vi "Main.vi"(11 "Module Admin":refnum<class "Delacor_lib_QMH_Module Admin.lvclass">) -> ()   [LabVIEW 2019, in "ContextHelp.lvlib"]
doc: "This template is based off of the Queued Message Handler design pattern and the Queued Message Handler project template that ships with LabVIEW.\n\nThe main difference is that the queue is private to this module and communication between modules is performed via Broadcast and Request events.\n\nRequest events are wrapped in public API methods and are handled in the Event Handling Loop (EHL) of this VI. Any module can register for Broadcast events sent by this module. The EHL generates messages based on user interface actions.\n\nThe Message Handling Loop (MHL) processes messages generated by the EHL, or by other messages. The messages are string values, so new messages can be added easily to the Message Cases case structure in the MHL. Each message cluster can also provide an optional value for Message Data, which is a variant that can be converted to whatever message-specific data is required.\n_____\nBased on DQMH Project Template 6.1.0.94.\n____\nPantherLAB Templates 1.0.0.5\nCopyright (c) 2022, PantherLAB"
uses:
  ContextHelp.lvlib
  <vilib>/Delacor/Delacor QMH/Libraries/Module Admin_class/Delacor_lib_QMH_Module Admin.lvclass
  Module Data--cluster.ctl
  <vilib>/Delacor/Delacor QMH/Libraries/Message Queue_class/Delacor_lib_QMH_Message Queue.lvclass/Delacor_lib_QMH_Message Queue.ctl
  Stop Argument--cluster.ctl
  <vilib>/Delacor/Delacor QMH/Libraries/Module Admin_class/Delacor_lib_QMH_Module Admin.lvclass/Delacor_lib_QMH_Module Admin.ctl
  Draw Panel Into Subpanel Argument--cluster.ctl
  Remove Panel from Subpanel Argument--cluster.ctl
  <vilib>/Delacor/Delacor QMH/Libraries/Message Queue_class/Delacor_lib_QMH_Enqueue Message (Single).vi
  <vilib>/Delacor/Delacor QMH/Libraries/Module Admin_class/Delacor_lib_QMH_Get External Launch.vi
  <vilib>/Utility/error.llb/Error Cluster From Error Code.vi
  <vilib>/ErrorRing/Error Ring.xnode
  <vilib>/Delacor/Delacor QMH/Libraries/Message Queue_class/Delacor_lib_QMH_Message Queue.lvclass
  Panther Dashboard/Panther Dashboard.lvlib
  Shared/Shared.lvlib
panel:
  out "Status":string
  out "error out":errorcluster
  in  "Edit Project Description":bool caption="Project Documentation"
  in  "Project Description":string
  in  "Edit Module Description":bool caption="Module Description"
  in  "Module Description":string
  in  "Edit VI":bool caption="Event Description"
  out "Event Connector Pane":picture
  in  "Event Description":string
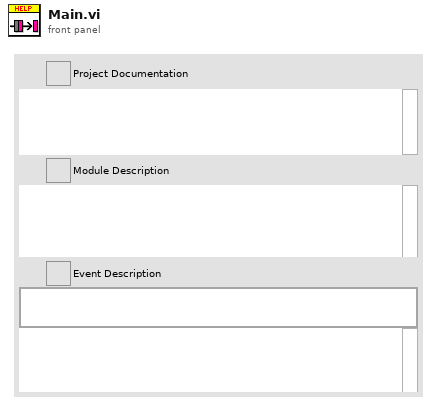
[diagram p1: front panel]
types:
  T1 = typedef "Panther Dashboard.lvlib/Broadcast Events--cluster.ctl" = cluster{"Module Did Init":refnum<user-event>, "Status Updated":refnum<user-event>, "Error Reported":refnum<user-event>, "Module Did Stop":refnum<user-event>, "Update Module Execution Status":refnum<user-event>, "References Updated":refnum<user-event>, "Projects Updated":refnum<user-event>, "Targets Updated":refnum<user-event>, "Progress updated":refnum<user-event>, "Scale Updated":refnum<user-event>, "Connector Pane Updated":refnum<user-event>, "Documentation Updated":refnum<user-event>, "Module Type Updated":refnum<user-event>, "Theme Updated":refnum<user-event>, "Project Description Updated":refnum<user-event>}
  T2 = typedef "ContextHelp.lvlib/Request Events--cluster.ctl" = cluster{"Stop Module":refnum<user-event>, "Show Panel":refnum<user-event>, "Hide Panel":refnum<user-event>, "Get Module Execution Status":refnum<user-event>, "Show Diagram":refnum<user-event>, "Wake up Helper Loop":refnum<user-event>, "Put Helper Loop to Sleep":refnum<user-event>, "Draw Panel Into Subpanel":refnum<user-event>, "Remove Panel from Subpanel":refnum<user-event>, "Refresh Panther Dashboard Broadcasts":refnum<user-event>}
  T3 = typedef "ContextHelp.lvlib/Module Data--cluster.ctl" = cluster{"Status":string, "SubPanel":refnum<vi>, "Panel Status":bool}
  T4 = enum8{"Enabled", "Disabled", "Disabled and Grayed Out"}
  T5 = enum32{"invalid lock state", "Not Locked", "Locked (No Password)", "Password-protected"}
  T6 = typedef "ContextHelp.lvlib/Stop Argument--cluster.ctl" = cluster{"Origin":string, "Exit via Stop Module Req?":bool, "Wait for Module to stop?":bool}
  T7 = typedef "ContextHelp.lvlib/Draw Panel Into Subpanel Argument--cluster.ctl" = cluster{"Sub Panel":refnum<vi>}
  T8 = typedef "ContextHelp.lvlib/Remove Panel from Subpanel Argument--cluster.ctl" = cluster{"Boolean":bool}
  T9 = enum32{"Invalid", "Standard", "Closed", "Hidden", "Minimized", "Maximized"}
  T10 = typedef "LVRectTypeDef.ctl" = cluster{"Left":i16, "Top":i16, "Right":i16, "Bottom":i16}
  T11 = typedef "Panther Dashboard.lvlib/Documentation--cluster.ctl" = cluster{"Module Description":string, "Event Description":string}
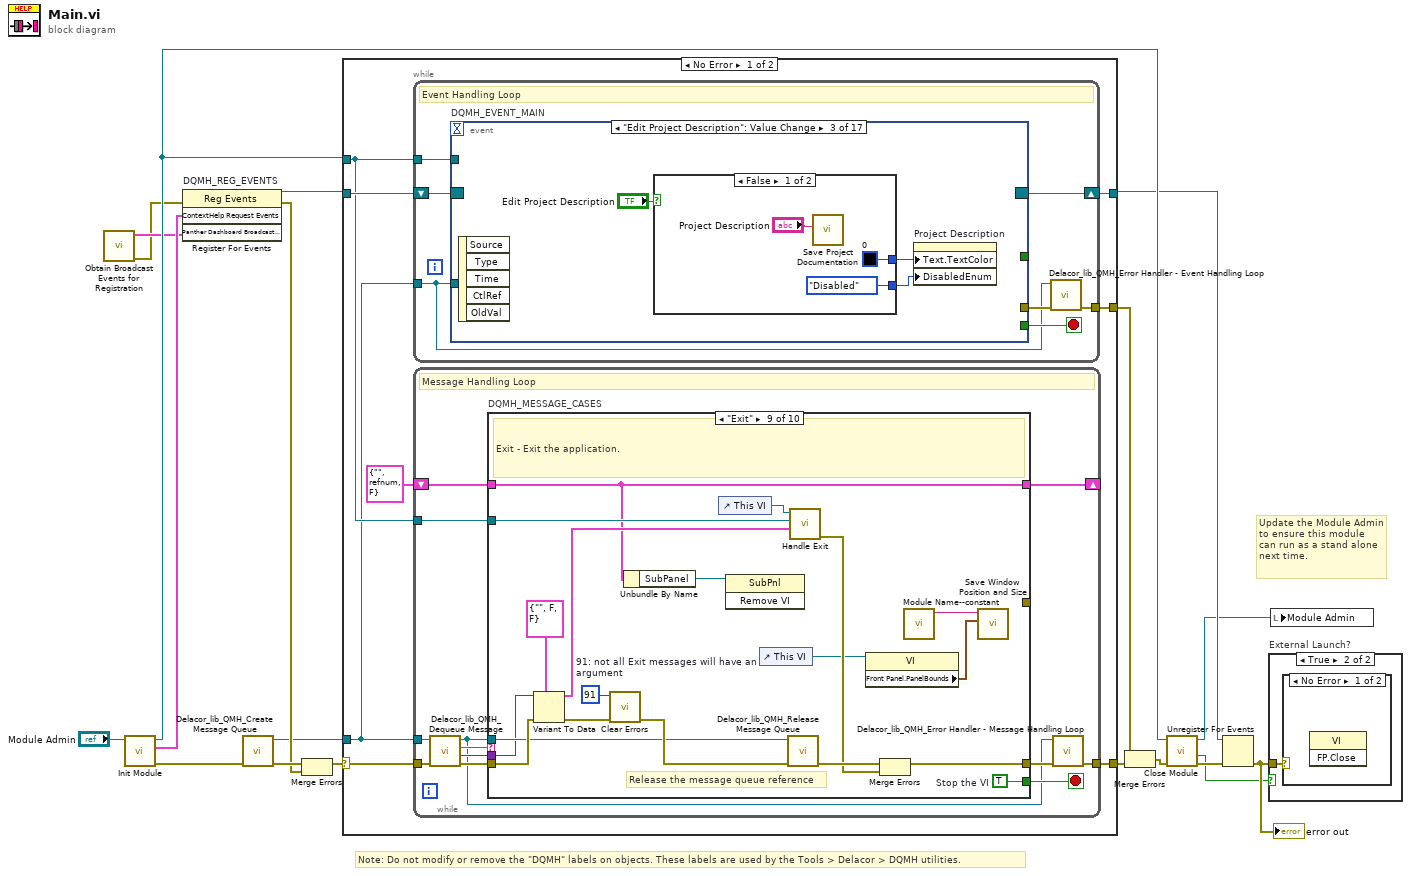
[diagram p0: block diagram]
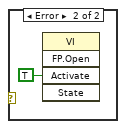
[diagram p3: hidden frame]
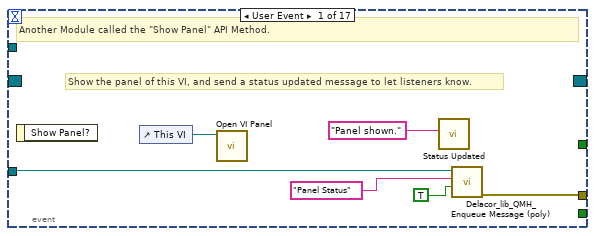
[diagram p4: hidden frame]
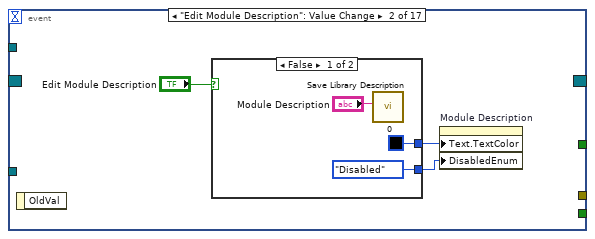
[diagram p5: hidden frame]
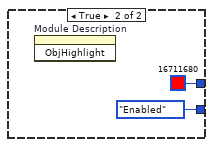
[diagram p6: hidden frame]
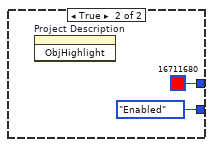
[diagram p7: hidden frame]
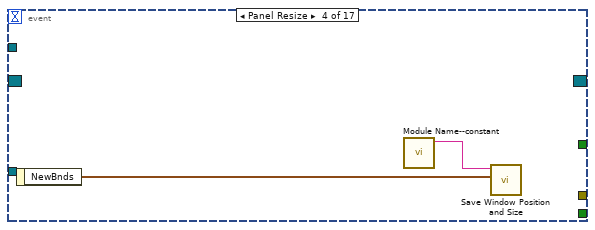
[diagram p8: hidden frame]
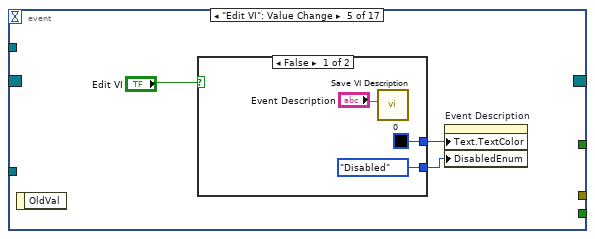
[diagram p9: hidden frame]
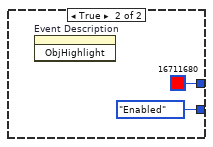
[diagram p10: hidden frame]
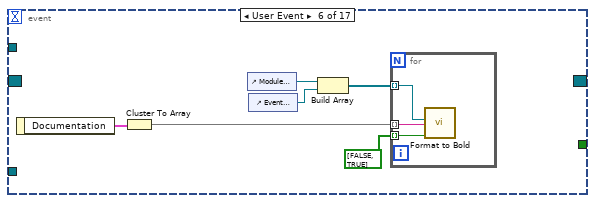
[diagram p11: hidden frame]
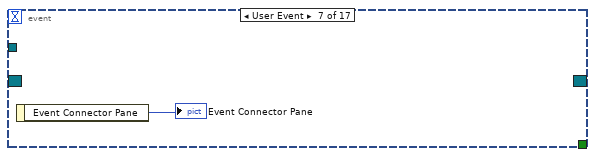
[diagram p12: hidden frame]
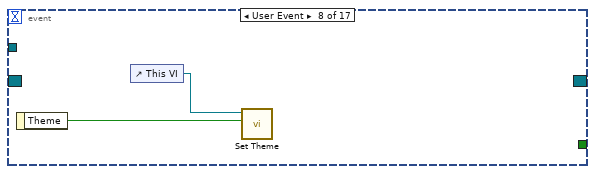
[diagram p13: hidden frame]
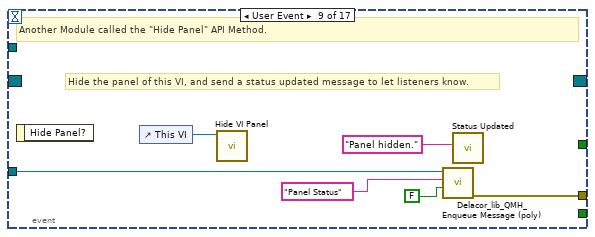
[diagram p14: hidden frame]
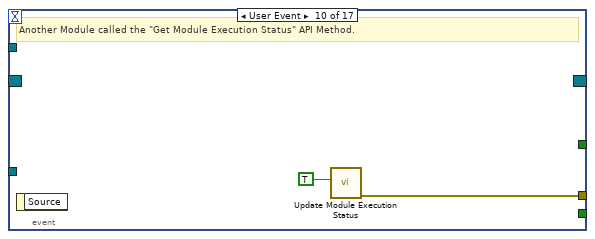
[diagram p15: hidden frame]
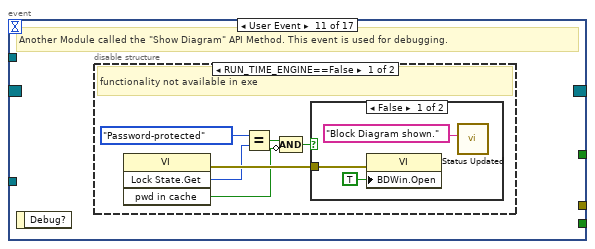
[diagram p16: hidden frame]
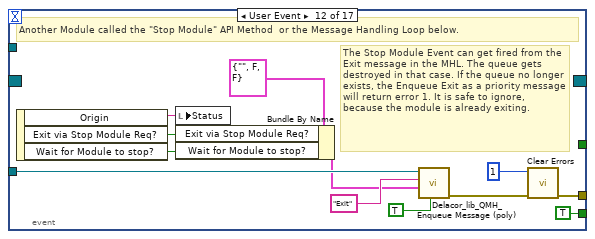
[diagram p19: hidden frame]
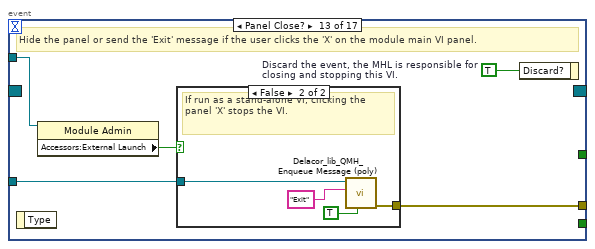
[diagram p20: hidden frame]
diagram:
  # "Note: Do not modify or remove the \"DQMH\" labels on objects. These labels are used by the Tools > Delacor > DQMH utilities."
  # "Update the Module Admin to ensure this module can run as a stand alone next time."
  n1 = call "Obtain Broadcast Events for Registration.vi"() -> ("error out"=w1:errorcluster, "Panther Dashboard Broadcast Events"=w2:T1)  [unwired: 9 in, 1 out]
  n2 = call "Init Module.vi"("Singleton Module Admin in"="Module Admin") -> ("error out"=w18:errorcluster, "ContextHelp Request Events"=w3:T2, "Singleton Module Admin out"=w10:refnum<class "Delacor_lib_QMH_Module Admin.lvclass">)  [unwired: 8 in]
  n3 = register-events "DQMH_REG_EVENTS"(error in=w1, w3, w2) -> (reference out=w8:refnum<event-registration>, error out=w11:errorcluster)  [unwired: 1 in]
  n4 = call <vilib>:"Delacor_lib_QMH_Create Message Queue.vi"("error in"=w18) -> ("error out"=w13:errorcluster, "Message Queue"=w7:refnum<class "Delacor_lib_QMH_Message Queue.lvclass">)  [unwired: 9 in]
  n5 = Merge Errors(w13, w11) -> (w12:errorcluster)
  n6 = case shown="No Error" w12 {
    selector: w12 -> [w25 w261]
    tunnel: [w27 w260] -> w19
    tunnel: [w24 w259] -> w9
    tunnel: w8 -> [w22 w259]
    tunnel: w7 -> [w20 w254]
    tunnel: [w26 _] -> w16
    tunnel: w10 -> [w21 w255]
    frame No Error {
      n7 = while {
        tunnel: w20 -> [w28]
        shift-right: [w31] -> w24
        shift-left: w22 -> [w32]
        tunnel: [w33] -> w26
        tunnel: w21 -> [w29]
        stop <- w30 stop-if-true
        # "Event Handling Loop"
        n8 = event "DQMH_EVENT_MAIN" shown="[2] \"Edit Project Description\": Value Change" {
          selector: w32 -> [_ _ _ _ _ _ _ _ _ _ _ _ _ _ _ w133 _]
          dyn-events: [_ _ _ _ _ _ _ _ _ _ _ _ _ _ _ w132 _] -> w31
          timeout: _ -> [_ _ _ _ _ _ _ _ _ _ _ _ _ _ _ _ _]
          tunnel: [_ _ _ _ _ _ _ _ _ _ _ TRUE ("Discard?") _ _ _ _ _] -> w30
          tunnel: w28 -> [w37 _ _ _ _ _ _ _ w79 _ _ w103 w110 w122 w128 _ _]
          tunnel: [w40 _ _ _ _ _ _ _ w84 w86 _ w106 w112 w123 w129 _ _] -> w34
          tunnel: w29 -> [_ _ _ _ _ _ _ _ _ _ _ _ w109 _ _ _ _]
          tunnel: [_ _ _ _ _ _ _ _ _ _ _ _ _ _ _ w130 _] -> _
          event User Event {
            # "Show the panel of this VI, and send a status updated message to let listeners know."
            # "Another Module called the \"Show Panel\" API Method."
            n9 = event-data() -> ()  [unwired: 1 in, 1 out]
            n10 = control-ref of="This VI"() -> (w39:refnum<vi>)
            n11 = call "Open VI Panel.vi"("VI"=w39) -> ()  [unwired: 10 in, 1 out]
            n12 = call "Status Updated.vi"("Status"="Panel shown." ("format string")) -> ()  [unwired: 10 in, 1 out]
            n13 = call-poly <vilib>:"Delacor_lib_QMH_Enqueue Message (poly).vi"("Message Data"=TRUE, "Message"="Panel Status" ("format string"), "Message Queue in"=w37) -> ("error out"=w40:errorcluster)  [unwired: 7 in, 1 out]
          }
          event "Edit Module Description": Value Change {
            n14 = event-data() -> ()  [unwired: 1 in, 1 out]
            n15 = case shown="False" "Edit Module Description" {
              tunnel: [u32 0 u32 16711680] -> w42
              tunnel: [T4."Disabled" ("Disabled") T4."Enabled" ("Disabled")] -> w43
              frame False {
                n16 = call "Save Library Description.vi"("Library Description"="Module Description") -> ()  [unwired: 10 in, 1 out]
              }
              frame True {
                n17 = invoke on="Module Description" class="Str" method="ObjHighlight"() -> ()  [unwired: 3 in, 3 out]
              }
            }
            n18 = property on="Module Description" class="Str"("Text.TextColor"=w42, "DisabledEnum"=w43) -> ()  [unwired: 2 in, 2 out]
          }
          event "Edit Project Description": Value Change {
            n19 = event-data() -> ()  [unwired: 1 in, 5 out]
            n20 = case shown="False" "Edit Project Description" {
              tunnel: [u32 0 u32 16711680] -> w50
              tunnel: [T4."Disabled" ("Disabled") T4."Enabled" ("Disabled")] -> w51
              frame False {
                n21 = call "Save Project Documentation.vi"("Project Description"="Project Description") -> ()  [unwired: 10 in, 1 out]
              }
              frame True {
                n22 = invoke on="Project Description" class="Str" method="ObjHighlight"() -> ()  [unwired: 3 in, 3 out]
              }
            }
            n23 = property on="Project Description" class="Str"("Text.TextColor"=w50, "DisabledEnum"=w51) -> ()  [unwired: 2 in, 2 out]
          }
          event Panel Resize {
            n24 = event-data() -> ("NewBnds"=w58:T10)  [unwired: 1 in]
            n25 = call "Module Name--constant.vi"() -> ("Module Name"=w57:string)  [unwired: 11 in]
            n26 = call "Save Window Position and Size.vi"("NewBnds"=w58, "Position Key"=w57) -> ()  [unwired: 9 in, 1 out]
          }
          event "Edit VI": Value Change {
            n27 = event-data() -> ()  [unwired: 1 in, 1 out]
            n28 = case shown="False" "Edit VI" {
              tunnel: [u32 0 u32 16711680] -> w60
              tunnel: [T4."Disabled" ("Disabled") T4."Enabled" ("Disabled")] -> w61
              frame False {
                n29 = call "Save VI Description.vi"("VI Description"="Event Description") -> ()  [unwired: 10 in, 1 out]
              }
              frame True {
                n30 = invoke on="Event Description" class="Str" method="ObjHighlight"() -> ()  [unwired: 3 in, 3 out]
              }
            }
            n31 = property on="Event Description" class="Str"("Text.TextColor"=w60, "DisabledEnum"=w61) -> ()  [unwired: 2 in, 2 out]
          }
          event User Event {
            n32 = event-data() -> ("Documentation"=w72:T11)  [unwired: 1 in]
            n33 = Cluster To Array(cluster=w72) -> (array=w70:string[])
            n34 = control-ref of="Module Description"() -> (w68:refnum<vi>)
            n35 = control-ref of="Event Description"() -> (w67:refnum<vi>)
            n36 = Build Array(w68, w67) -> (w69:refnum<vi>[])
            n37 = for {
              tunnel: bool[] [FALSE, TRUE] ("Adjust Height?") -> [w75] mode=indexing
              tunnel: w70 -> [w74] mode=indexing
              tunnel: w69 -> [w73] mode=indexing
              n38 = call "Format to Bold.vi"("Adjust Height?"=w75, "String Value"=w74, "String Ref"=w73) -> ()  [unwired: 9 in]
            }
          }
          event User Event {
            n39 = event-data() -> ("Event Connector Pane"=→"Event Connector Pane":picture)  [unwired: 1 in]
          }
          event User Event {
            n40 = event-data() -> ("Theme"=w77:bool)  [unwired: 1 in]
            n41 = control-ref of="This VI"() -> (w78:refnum<vi>)
            n42 = call "Set Theme.vi"("Dark?"=w77, "VI in"=w78) -> ()  [unwired: 10 in]
          }
          event User Event {
            # "Hide the panel of this VI, and send a status updated message to let listeners know."
            # "Another Module called the \"Hide Panel\" API Method."
            n43 = event-data() -> ()  [unwired: 1 in, 1 out]
            n44 = control-ref of="This VI"() -> (w83:refnum<vi>)
            n45 = call "Hide VI Panel.vi"("VI"=w83) -> ()  [unwired: 10 in, 1 out]
            n46 = call-poly <vilib>:"Delacor_lib_QMH_Enqueue Message (poly).vi"("Message Data"=FALSE, "Message"="Panel Status" ("format string"), "Message Queue in"=w79) -> ("error out"=w84:errorcluster)  [unwired: 7 in, 1 out]
            n47 = call "Status Updated.vi"("Status"="Panel hidden." ("format string")) -> ()  [unwired: 10 in, 1 out]
          }
          event User Event {
            # "Another Module called the \"Get Module Execution Status\" API Method."
            n48 = event-data() -> ()  [unwired: 1 in, 1 out]
            n49 = call "Update Module Execution Status.vi"("Running?"=TRUE) -> ("error out"=w86:errorcluster)  [unwired: 10 in]
          }
          event User Event {
            # "Another Module called the \"Show Diagram\" API Method. This event is used for debugging."
            n50 = event-data() -> ()  [unwired: 1 in, 1 out]
            n51 = disable-structure shown="RUN_TIME_ENGINE==False" {
              frame condition #0 (active) {
                # "functionality not available in exe"
                n52 = invoke class="VI" method="Lock State.Get"() -> (error out=w92:errorcluster, "Get Lock State"=w91:T5, "pwd in cache"=w88:bool)  [unwired: 4 in, 1 out]
                n53 = Equal?(x=T5."Password-protected", y=w91) -> (x = y?=w89:bool)
                n54 = Compound Arithmetic op=AND(w89, invert w88) -> (w87:bool)
                n55 = case shown="False" w87 {
                  tunnel: w92 -> [w95 _]
                  frame False {
                    n56 = property class="VI"(error in=w95, "BDWin.Open"=TRUE ("Block Diagram Window:Open")) -> ()  [unwired: 1 in, 2 out]
                    n57 = call "Status Updated.vi"("Status"="Block Diagram shown." ("format string")) -> ()  [unwired: 10 in, 1 out]
                  }
                  frame True {
                    # "Password-protected VI, and the password is not in the cache. Do not show the diagram."
                  }
                }
              }
              frame condition #1 {
              }
            }
          }
          event User Event {
            # "The Stop Module Event can get fired from the Exit message in the MHL. The queue gets destroyed in that case. If the queue no longer exists, the Enqueue Exit as a priority message will return error 1. It is safe to ignore, because the module is already exiting."
            # "Another Module called the \"Stop Module\" API Method  or the Message Handling Loop below."
            n58 = event-data() -> ("Origin"=w102:string, "Exit via Stop Module Req?"=w98:bool, "Wait for Module to stop?"=w97:bool)  [unwired: 1 in]
            n59 = local write "Status"(w102) -> ()
            n60 = Bundle By Name(cluster=T6 {"Origin"="", "Exit via Stop Module Req?"=FALSE, "Wait for Module to stop?"=FALSE} ("Stop Argument"), "Exit via Stop Module Req?"=w98, "Wait for Module to stop?"=w97) -> (w96:T6)
            n61 = call-poly <vilib>:"Delacor_lib_QMH_Enqueue Message (poly).vi"("Priority Message? (F)"=TRUE, "Message Data"=w96, "Message"="Exit", "Message Queue in"=w103) -> ("error out"=w107:errorcluster)  [unwired: 6 in, 1 out]
            n62 = call <vilib>:"Clear Errors.vi"("error in (no error)"=w107, "specific error code to clear (0: all)"=1) -> ("error out"=w106:errorcluster)  [unwired: 4 in, 1 out]
          }
          event Panel Close? {
            w111 = TRUE  # Discard the event, the MHL is responsible for closing and stopping this VI.
            # "Hide the panel or send the 'Exit' message if the user clicks the 'X' on the module main VI panel."
            n63 = event-data() -> ()  [unwired: 1 in, 1 out]
            n64 = property class="Module Admin"(reference=w109) -> ("Accessors:External Launch"=w108:bool)  [unwired: 1 in, 2 out]
            n65 = case shown="False" w108 {
              tunnel: w110 -> [_ w116]
              tunnel: [_ w117] -> w112
              frame True {
                # "If externally launched, clicking the 'X' hides the panel, but doesn't close it."
                n66 = control-ref of="This VI"() -> (w113:refnum<vi>)
                n67 = call "Hide VI Panel.vi"("VI"=w113) -> ()  [unwired: 10 in, 1 out]
              }
              frame False {
                # "If run as a stand-alone VI, clicking the panel 'X' stops the VI."
                n68 = call-poly <vilib>:"Delacor_lib_QMH_Enqueue Message (poly).vi"("Priority Message? (F)"=TRUE, "Message"="Exit", "Message Queue in"=w116) -> ("error out"=w117:errorcluster)  [unwired: 7 in, 1 out]
              }
            }
            n69 = event-data("Discard?"=w111) -> ()  [unwired: 1 in, 1 out]
          }
          event User Event {
            # "Another Module called the \"Draw your Panel into Subpanel\" API Method."
            n70 = event-data() -> ("Sub Panel"=w118:refnum<vi>)  [unwired: 1 in]
            n71 = Bundle(cluster=T7 {"Sub Panel"=refnum} ("Draw your Panel into Subpanel Argument"), "Sub Panel"=w118) -> (w119:T7)
            n72 = call-poly <vilib>:"Delacor_lib_QMH_Enqueue Message (poly).vi"("Message Data"=w119, "Message"="Draw Panel into Subpanel", "Message Queue in"=w122) -> ("error out"=w123:errorcluster)  [unwired: 7 in, 1 out]
          }
          event User Event {
            # "Another Module called the \"Remove Panel from Subpanel\" API Method."
            n73 = event-data() -> ("Boolean"=w124:bool)  [unwired: 1 in]
            n74 = Bundle(cluster=T8 {"Boolean"=FALSE} ("Remove Panel from Subpanel Argument"), "Boolean"=w124) -> (w125:T8)
            n75 = call-poly <vilib>:"Delacor_lib_QMH_Enqueue Message (poly).vi"("Message Data"=w125, "Message"="Remove Panel from Subpanel", "Message Queue in"=w128) -> ("error out"=w129:errorcluster)  [unwired: 7 in, 1 out]
          }
          event User Event {
            # "Another Module called the \"Refresh Panther Dashboard Broadcasts\" API Method."
            n76 = event-data() -> ()  [unwired: 1 in, 1 out]
            n77 = call "Obtain Broadcast Events for Registration.vi"() -> ("Already running?"=w130:bool, "Panther Dashboard Broadcast Events"=w131:T1)  [unwired: 9 in, 1 out]
            n78 = register-events "Refresh Panther Broadcasts"(reference=w133, w131) -> (reference out=w132:refnum<event-registration>)  [unwired: 2 in, 1 out]
          }
          event User Event {
            n79 = event-data() -> ("Project Description"=w134:string)  [unwired: 1 in]
            n80 = local write "Project Description"(w134) -> ()
          }
        }
        n81 = call-dynamic "Delacor_lib_QMH_Error Handler - Event Handling Loop.vi"("error in"=w34, "Message Queue in"=w28) -> ("dup error in"=w33:errorcluster)  [unwired: 8 in, 1 out]
      }
      n82 = while {
        tunnel: w20 -> [w137]
        shift-right: [w141] -> _
        shift-left: T3 {"Status"="", "SubPanel"=refnum, "Panel Status"=FALSE} ("Data Cluster") -> [w142]
        tunnel: w25 -> [w145]
        tunnel: [w143] -> w27
        tunnel: w21 -> [w135]
        stop <- w140 stop-if-true
        # "Message Handling Loop"
        n83 = call-dynamic "Delacor_lib_QMH_Dequeue Message.vi"("error in"=w145, "Message Queue in"=w137) -> ("error out"=w144:errorcluster, "Message Data"=w138:variant, "Message"=w139:string, "Message Queue out"=w136:refnum<class "Delacor_lib_QMH_Message Queue.lvclass">)  [unwired: 6 in]
        n84 = case "DQMH_MESSAGE_CASES" shown="\"Exit\"" w139 {
          selector: w139 -> [_ _ _ _ _ _ _ _ _ w241]
          tunnel: w136 -> [_ _ _ _ _ _ _ w207 w233 _]
          tunnel: w144 -> [w166 w170 w181 w190 w199 w202 w204 w214 w239 w243]
          tunnel: [w164 w170 w179 w189 w198 w201 w204 w210 w236 w244] -> w146
          tunnel: w142 -> [w155 w169 w178 w185 w197 w200 w203 w209 w225 w242]
          tunnel: [w154 w169 w172 w185 w194 w200 w203 w209 w225 w242] -> w141
          tunnel: [_ _ _ _ _ _ _ _ w232 _] -> w140
          tunnel: w138 -> [_ _ w177 w187 w196 _ _ w208 w231 _]
          tunnel: w135 -> [w156 _ _ _ _ _ _ w206 w226 _]
          tunnel: [w163 _ _ _ _ _ _ _ _ _] -> _
          frame "Initialize" {
            w150 = "Initial Message" ("Initial Message")
            # "Initialize - Any operation that needs to be done before the module can receive messages. Synchronize Caller Events.vi will inform Start Module.vi that the module has launched and is ready to receive messages. Module Did Init.vi will broadcast that the module initialized."
            n85 = call "Synchronize Caller Events.vi"("error in (no error)"=w166, "Singleton Module Admin in"=w156) -> ("error out"=w165:errorcluster, "Singleton Module Admin out"=w151:refnum<class "Delacor_lib_QMH_Module Admin.lvclass">)  [unwired: 8 in]
            n86 = property class="Module Admin"(reference=w151) -> ("Accessors:External Launch"=w160:bool)  [unwired: 1 in, 2 out]
            n87 = call "Module Name--constant.vi"() -> ("Module Name"=w148:string)  [unwired: 11 in]
            n88 = control-ref of="This VI"() -> (w149:refnum<vi>)
            n89 = Select(t=T9."Hidden" ("State"), s=w160, f=T9."Standard" ("State")) -> (s? t:f=w157:T9)
            n90 = property class="VI"("Front Panel.Title"="DQMH Project Context Help" ("Front Panel Window:Title")) -> (reference out=w162:refnum<vi>, error out=w168:errorcluster)  [unwired: 2 in]
            n91 = call "Read Window Position and Size.vi"("Position Key"=w148, "VI Refnum"=w149) -> ("error out"=w163:errorcluster)  [unwired: 9 in]
            n92 = call "Module Name--constant.vi"() -> ("Module Name"=w152:string)  [unwired: 11 in]
            n93 = invoke class="VI" method="FP.Open"(reference=w162, error in=w168, "State"=w157) -> (reference out=w161:refnum<vi>, error out=w167:errorcluster)  [unwired: 2 in, 3 out]
            n94 = call "Module Did Init.vi"("error in (no error)"=w165, "Initialized?"=TRUE, "Origin"=w152) -> ("error out"=w164:errorcluster)  [unwired: 8 in]
            n95 = Bundle By Name(cluster=w155, "Status"=w150) -> (w154:T3)
            n96 = invoke class="VI" method="FP.Center"(reference=w161, error in=w167) -> ()  [unwired: 1 in, 3 out]
            "Status" <- w150
          }
          frame "---Module Specific---" {
            # "Separator -- The following cases handle messages specific to this Module."
          }
          frame "Draw Panel into Subpanel" {
            # "#PantherLAB_How_To\nThis module request allows to draw Main.vi into any \nsubpanel provided"
            # "Request made to the module to draw itself into a subpanel provided"
            n97 = Variant To Data(error in=w181, type=T7 {"Sub Panel"=refnum} ("Draw your Panel into Subpanel Argument"), Variant=w177) -> (data=w175:T7, error out=w180:errorcluster)
            n98 = Unbundle By Name(w175) -> ("Sub Panel"=w173:refnum<vi>)
            n99 = control-ref of="This VI"() -> (w174:refnum<vi>)
            n100 = call "Draw Panel Into Subpanel Procedure.vi"("error in"=w180, "SubPanel in"=w173, "This VI"=w174) -> ("error out"=w179:errorcluster, "SubPanel out"=w171:refnum<vi>)  [unwired: 7 in]
            n101 = Bundle By Name(cluster=w178, "SubPanel"=w171) -> (w172:T3)
          }
          frame "Remove Panel from Subpanel" {
            # "Request to the module to remove itself from the subpanel"
            n102 = Variant To Data(error in=w190, type=T8 {"Boolean"=FALSE} ("Remove Panel from Subpanel Argument"), Variant=w187) -> (error out=w189:errorcluster)  [unwired: 1 out]
            n103 = Unbundle By Name(w185) -> ("Panel Status"=w183:bool, "SubPanel"=w184:refnum<vi>)
            n104 = invoke class="SubPnl" method="Remove VI"(reference=w184) -> (error out=w188:errorcluster)  [unwired: 2 in, 2 out]
            n105 = control-ref of="This VI"() -> (w182:refnum<vi>)
            n106 = case shown="False" w183 {
              tunnel: w188 -> [_ _]
              tunnel: w182 -> [w191 w192]
              frame False {
                # "Hiden"
                n107 = call "Hide VI Panel.vi"("VI"=w191) -> ()  [unwired: 10 in, 1 out]
              }
              frame True {
                # "Visible"
                n108 = call "Open VI Panel.vi"("VI"=w192) -> ()  [unwired: 10 in, 1 out]
              }
            }
          }
          frame "Panel Status" {
            n109 = Variant To Data(error in=w199, type=TRUE, Variant=w196) -> (data=w193:bool, error out=w198:errorcluster)
            n110 = Bundle By Name(cluster=w197, "Panel Status"=w193) -> (w194:T3)
          }
          frame "---Copy This Frame---" {
            # "Duplicate this frame when creating new messages.  Change this comment in the duplicated frame to describe this message."
            n111 = Merge Errors(w202) -> (w201:errorcluster)
          }
          frame "---Exit and Error Handling---" {
            # "Separator - The following cases handle errors and exit messages."
          }
          frame "Error" {
            # "#CodeRecommended - If you ever change the name of this \"Error\" message, you'll need to update the name in the Check Loop Error.vi as well."
            # "#CodeRecommended - If the module is running in standalone mode (External Launch = FALSE), this code will pop up an error dialog and call the 'Exit' message if an error occurs. Add more fine-grained error handling here."
            # "Error - Check the error message data and respond accordingly. This message is sent by the \"Error Handler\" VIs at the end of each loop in this application."
            n112 = property class="Module Admin"(reference=w206) -> ("Accessors:External Launch"=w205:bool)  [unwired: 1 in, 2 out]
            n113 = Variant To Data(error in=w214, type=errorcluster {"status"=FALSE, "code"=0, "source"=""} ("error constant"), Variant=w208) -> (data=w215:errorcluster, error out=w212:errorcluster)
            n114 = call "Error Reported.vi"("Error"=w215) -> ()  [unwired: 10 in, 1 out]
            n115 = case shown="False" w205 {
              tunnel: [w220 _] -> w211
              tunnel: w207 -> [w218 _]
              tunnel: w215 -> [w219 _]
              frame False {
                # "If the module is running standalone, then pop up an error dialog and call the \"Exit\" message."
                n116 = call <vilib>:"Simple Error Handler.vi"("error in (no error)"=w219) -> ()  [unwired: 4 in, 5 out]
                n117 = call-poly <vilib>:"Delacor_lib_QMH_Enqueue Message (poly).vi"("Priority Message? (F)"=TRUE, "Message"="Exit", "Message Queue in"=w218) -> ("error out"=w220:errorcluster)  [unwired: 7 in, 1 out]
              }
              frame True {
                # "If the module was launched externally, calling the Error Reported broadcast VI is the only action performed by the \"Error\" message. The module's caller can then process the error appropriately."
              }
            }
            n118 = Merge Errors(w212, w211) -> (w210:errorcluster)
            n119 = local write "error out"(w210) -> ()
          }
          frame "Exit" {
            w230 = 91  # 91: not all Exit messages will have an argument
            w232 = TRUE  # Stop the VI
            # "Release the message queue reference"
            # "Exit - Exit the application."
            n120 = Variant To Data(error in=w239, type=T6 {"Origin"="", "Exit via Stop Module Req?"=FALSE, "Wait for Module to stop?"=FALSE} ("Stop Argument"), Variant=w231) -> (data=w228:T6, error out=w235:errorcluster)
            n121 = call <vilib>:"Clear Errors.vi"("error in (no error)"=w235, "specific error code to clear (0: all)"=w230) -> ("error out"=w238:errorcluster)  [unwired: 4 in, 1 out]
            n122 = Unbundle By Name(w225) -> ("SubPanel"=w224:refnum<vi>)
            n123 = control-ref of="This VI"() -> (w227:refnum<vi>)
            n124 = invoke class="SubPnl" method="Remove VI"(reference=w224) -> ()  [unwired: 2 in, 3 out]
            n125 = control-ref of="This VI"() -> (w223:refnum<vi>)
            n126 = call-dynamic "Delacor_lib_QMH_Release Message Queue.vi"("error in"=w238, "Message Queue"=w233) -> ("error out"=w237:errorcluster)  [unwired: 9 in]
            n127 = call "Handle Exit.vi"("Stop Argument"=w228, "Admin in"=w226, "VI reference"=w227) -> ("error out"=w234:errorcluster)  [unwired: 7 in, 1 out]
            n128 = property class="VI"(reference=w223) -> ("Front Panel.PanelBounds"=w222:T10)  [unwired: 1 in, 2 out]
            n129 = Merge Errors(w237, w234) -> (w236:errorcluster)
            n130 = call "Module Name--constant.vi"() -> ("Module Name"=w221:string)  [unwired: 11 in]
            n131 = call "Save Window Position and Size.vi"("NewBnds"=w222, "Position Key"=w221) -> ()  [unwired: 9 in, 1 out]
          }
          frame Default {
            # "'Default' case only runs if there is a message that isn't defined in any of the other cases.  Output a programming error."
            n132 = call "Module Name--constant.vi"() -> ("Module Name"=w240:string)  [unwired: 11 in]
            n133 = xnode "Error Ring"("parameter 0"=w241, "parameter 1"=w240) -> ("error out"=w245:errorcluster)
            n134 = Merge Errors(w243, w245) -> (w244:errorcluster)
          }
        }
        n135 = call-dynamic "Delacor_lib_QMH_Error Handler - Message Handling Loop.vi"("error in"=w146, "Message Queue in"=w136) -> ("dup error in"=w143:errorcluster)  [unwired: 8 in, 1 out]
      }
    }
    frame Error {
      # "Synchronize Caller Events.vi will inform Start Module.vi that the module has launched and will let the code calling Start Module.vi register for broadcasts and would permit the caller receive the broadcast that an error occurred at launch time."
      n136 = call-dynamic "Delacor_lib_QMH_Release Message Queue.vi"("error in"=w261, "Message Queue"=w254) -> ("error out"=w260:errorcluster)  [unwired: 9 in]
      n137 = call "Synchronize Caller Events.vi"("Singleton Module Admin in"=w255) -> ("error out"=w262:errorcluster)  [unwired: 9 in, 1 out]
      n138 = call "Module Name--constant.vi"() -> ("Module Name"=w258:string)  [unwired: 11 in]
      n139 = Format Into String(format string="An error occurred during initialization. %s is no longer running.", w258) -> (resulting string=w256:string)  [unwired: 2 in, 1 out]
      n140 = Merge Errors(w260, w262) -> (w263:errorcluster)
      n141 = call "Error Reported.vi"("Additional Information"=w256, "Error"=w263) -> ()  [unwired: 9 in, 1 out]
    }
  }
  n142 = Merge Errors(w16, w19) -> (w15:errorcluster)
  n143 = call "Close Module.vi"("error in (no error)"=w15, "Module Admin in"=w10) -> ("error out"=w17:errorcluster, "External Launch"=w4:bool, "Module Admin out"=w5:refnum<class "Delacor_lib_QMH_Module Admin.lvclass">)  [unwired: 7 in]
  n144 = Unregister For Events(event registration refnum=w9, error in=w17) -> (error out=w14:errorcluster)
  "error out" <- w14
  n145 = case "External Launch?" shown="True" w4 {
    tunnel: w14 -> [_ w264]
    frame False {
    }
    frame True {
      n146 = case shown="No Error" w264 {
        frame No Error {
          n147 = invoke class="VI" method="FP.Close"() -> ()  [unwired: 3 in, 3 out]
        }
        frame Error {
          n148 = invoke class="VI" method="FP.Open"("Activate"=TRUE ("Activate?")) -> ()  [unwired: 4 in, 5 out]
        }
      }
    }
  }
  n149 = local write "Module Admin"(w5) -> ()
